vi "Cleanup.vi"(8 "error in (no error)":errorcluster, 11 "Sequence in":refnum<class "Sequence.lvclass">) -> (0 "error out":errorcluster)   [LabVIEW 2020, in "VolatusSeq.lvlib" / "Sequence.lvclass"]
uses:
  Sequence.lvclass
  Sequence.lvclass/Sequence.ctl
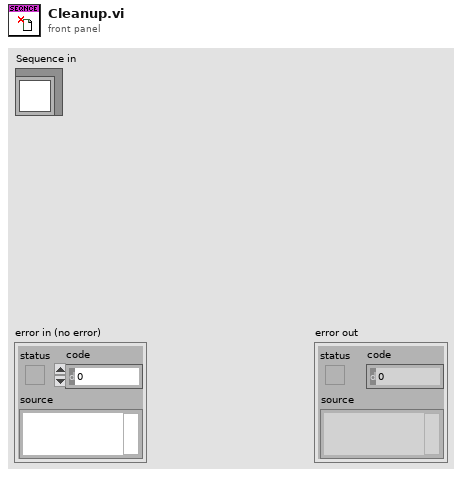
[diagram p1: front panel]
types:
  T1 = typedef "VolatusSeq.lvlib/State Control.ctl" = cluster{"State":refnum<notifier>, "Time":refnum<notifier>, "Request State":refnum<notifier>, "Abort":refnum<notifier>, "Reset":refnum<notifier>, "Close":refnum<notifier>, "Vars SEQ":refnum<queue>}
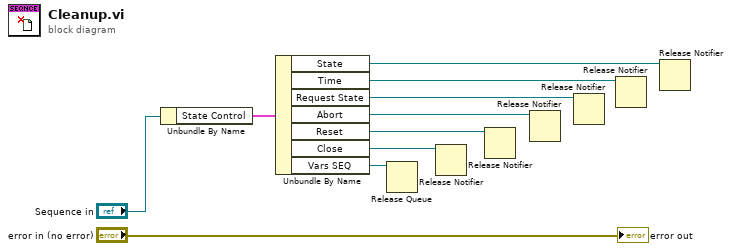
[diagram p0: block diagram]
diagram:
  n1 = Unbundle By Name("Sequence in") -> ("State Control"=w8:T1)
  n2 = Unbundle By Name(w8) -> ("State"=w3:refnum<notifier>, "Time"=w4:refnum<notifier>, "Request State"=w5:refnum<notifier>, "Abort"=w6:refnum<notifier>, "Reset"=w7:refnum<notifier>, "Close"=w2:refnum<notifier>, "Vars SEQ"=w1:refnum<queue>)
  n3 = Release Queue(queue=w1) -> ()  [unwired: 2 in, 3 out]
  n4 = Release Notifier(notifier=w2) -> ()  [unwired: 2 in, 3 out]
  n5 = Release Notifier(notifier=w7) -> ()  [unwired: 2 in, 3 out]
  n6 = Release Notifier(notifier=w6) -> ()  [unwired: 2 in, 3 out]
  n7 = Release Notifier(notifier=w5) -> ()  [unwired: 2 in, 3 out]
  n8 = Release Notifier(notifier=w4) -> ()  [unwired: 2 in, 3 out]
  n9 = Release Notifier(notifier=w3) -> ()  [unwired: 2 in, 3 out]
  "error out" <- "error in (no error)"
